vi "get file and start.vi"() -> (0 "file path":path, 3 "start time":u32, 4 "canceled":bool)   [LabVIEW 2012]
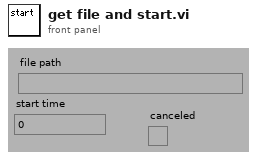
[diagram p1: front panel]
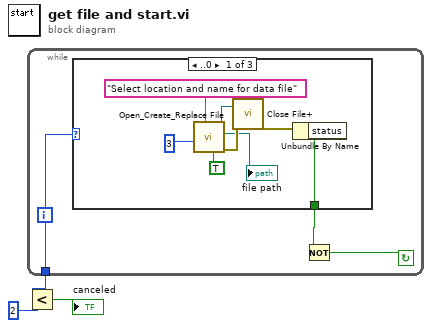
[diagram p0: block diagram]
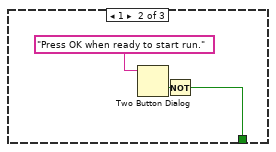
[diagram p2: hidden frame]
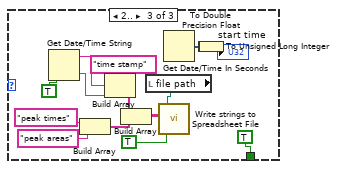
[diagram p3: hidden frame]
diagram:
  n1 = while {
    tunnel: [w6] -> w3
    i -> [w6]
    stop <- w5 continue-if-true
    n2 = case shown="..0" w6 {
      tunnel: [w8 w15 TRUE] -> w4
      frame ..0 {
        n3 = call <vilib>:"Open_Create_Replace File.vi"("advisory dialog? (display:T)"=TRUE, "prompt"="Select location and name for data file", "function (open:0)"=3) -> ("error out"=w10:errorcluster, "new file path"=→"file path":path, "refnum"=w11:refnum<file>)  [unwired: 5 in, 1 out]
        n4 = call <vilib>:"Close File+.vi"("error in (no error)"=w10, "refnum"=w11) -> ("error out"=w14:errorcluster)  [unwired: 3 in, 2 out]
        n5 = Unbundle By Name(w14) -> ("status"=w8:bool)
      }
      frame 1 {
        n6 = Two Button Dialog(message="Press OK when ready to start run.") -> (T button?=w16:bool)  [unwired: 2 in]
        n7 = Not(x=w16) -> (.not. x?=w15:bool)
      }
      frame 2.. {
        n8 = Get Date/Time String(want seconds? (F)=TRUE) -> (date string=w25:string, time string=w26:string)  [unwired: 2 in]
        n9 = Build Array("peak times", "peak areas") -> (w28:string[])
        n10 = Build Array("time stamp", w25, w26) -> (w29:string[])
        n11 = Build Array(w29, w28) -> (w27:string[][])
        n12 = local read "file path"() -> (w22:path)
        n13 = call "Write strings to Spreadsheet File.vi"("append to file? (new file:F)"=TRUE, "2D data"=w27, "file path (dialog if empty)"=w22) -> ()  [unwired: 5 in, 1 out]
        n14 = Get Date/Time In Seconds() -> (seconds since 1Jan1904=w18:timestamp)
        n15 = To Double Precision Float(number=w18) -> (double precision float=w19:dbl)
        n16 = To Unsigned Long Integer(number=w19) -> (unsigned 32bit integer=→"start time":u32)
      }
    }
    n17 = Not(x=w4) -> (.not. x?=w5:bool)
  }
  n18 = Less?(x=w3, y=2) -> (x < y?=→"canceled":bool)
